vi "Coord window-Sanity check coord list.vi"(8 "error in (no error)":errorcluster) -> (0 "error out":errorcluster, 3 "Discard":bool)   [LabVIEW 2013]
uses:
  Globals/Coord window-Globals.vi
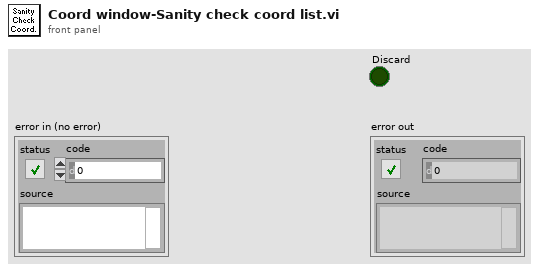
[diagram p1: front panel]
types:
  T1 = typedef "Coordinate list window refs.ctl" = cluster{"Window Name (i.e. Key)":string, "menu reference":refnum<k9>, "VI's reference":refnum<vi>, "Pane 1":refnum<vi>, "Pane 2":refnum<vi>, "Coord Listbox":refnum<vi>, "File name":refnum<vi>, "Picture Map":refnum<vi>, "Stage XYZ Position ind.":refnum<vi>}
  T2 = typedef "LVBoundsTypeDef.ctl" = cluster{"Width":u32, "Height":u32}
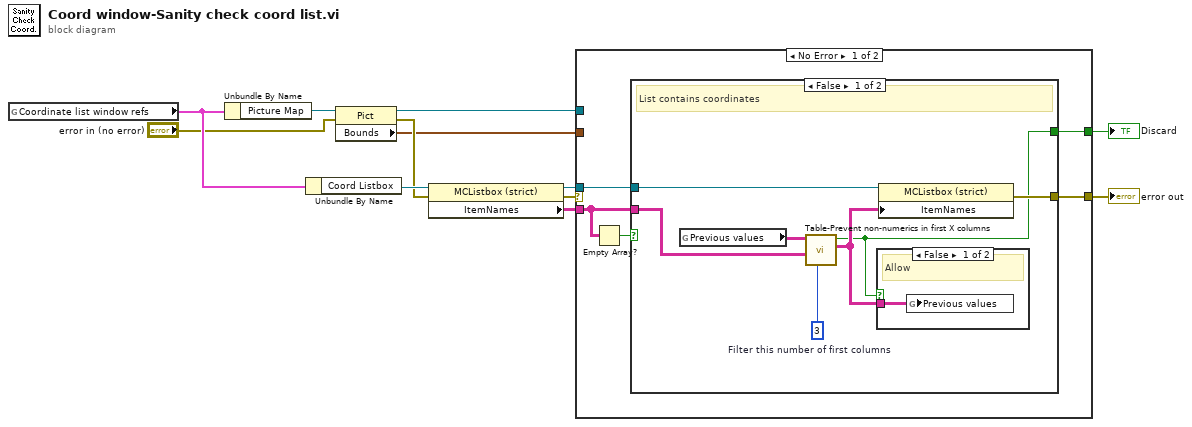
[diagram p0: block diagram]
diagram:
  n1 = global read "Coord window-Globals.vi" "Coordinate list window refs"() -> (w2:T1)
  n2 = Unbundle By Name(w2) -> ("Picture Map"=w10:refnum<vi>)
  n3 = Unbundle By Name(w2) -> ("Coord Listbox"=w12:refnum<vi>)
  n4 = property on="Property Node" class="Pict"(reference=w10, error in="error in (no error)") -> (reference out=w9:refnum<vi>, error out=w8:errorcluster, "Bounds"=w7:T2)
  n5 = property on="Property Node" class="MCListbox (strict)"(reference=w12, error in=w8) -> (reference out=w4:refnum<vi>, error out=w6:errorcluster, "ItemNames"=w11:string[][])
  n6 = case shown="No Error" w6 {
    selector: w6 -> [_ w26]
    tunnel: w11 -> [w17 _]
    tunnel: w9 -> [_ _]
    tunnel: w7 -> [_ _]
    tunnel: [w14 w26] -> w5
    tunnel: w4 -> [w15 _]
    tunnel: [w13 _] -> w3
    frame No Error {
      n7 = Empty Array?(array=w17) -> (empty?=w16:bool)
      n8 = case shown="False" w16 {
        tunnel: w17 -> [w21 _]
        tunnel: w15 -> [w23 _]
        tunnel: [w22 _] -> w14
        tunnel: [w18 _] -> w13
        frame False {
          w19 = 3  # Filter this number of first columns
          # "List contains coordinates"
          n9 = global read "Coord window-Globals.vi" "Previous values"() -> (w20:string[][])
          n10 = call "Table-Prevent non-numerics in first X columns.vi"("Filter this number of first columns"=w19, "New Value in"=w21, "Old Value in"=w20) -> ("Filtered array"=w24:string[][], "Discard"=w18:bool)  [unwired: 6 in, 1 out]
          n11 = case shown="False" w18 {
            tunnel: w24 -> [w25 _]
            frame False {
              # "Allow"
              n12 = global write "Coord window-Globals.vi" "Previous values"(w25) -> ()
            }
            frame True {
              # "Discard"
            }
          }
          n13 = property on="Property Node" class="MCListbox (strict)"(reference=w23, "ItemNames"=w24) -> (error out=w22:errorcluster)  [unwired: 1 in, 1 out]
        }
        frame True {
          # "List is empty"
        }
      }
    }
    frame Error {
    }
  }
  "error out" <- w5
  "Discard" <- w3
